vi "niFpgaMemoryEmulationDramWriteAndRequestData.vi"(0 "address":u32, 1 "name":string, 2 "number of elements":u32, 3 "fifo size":u32, 5 "data":i32, 7 "write":bool, 9 "input valid":bool, 11 "error in (no error)":errorcluster, 12 "byte enables":i64, 13 "ref in wired":bool) -> (10 "ready for input":bool, 15 "error out":errorcluster)   [LabVIEW 2017]
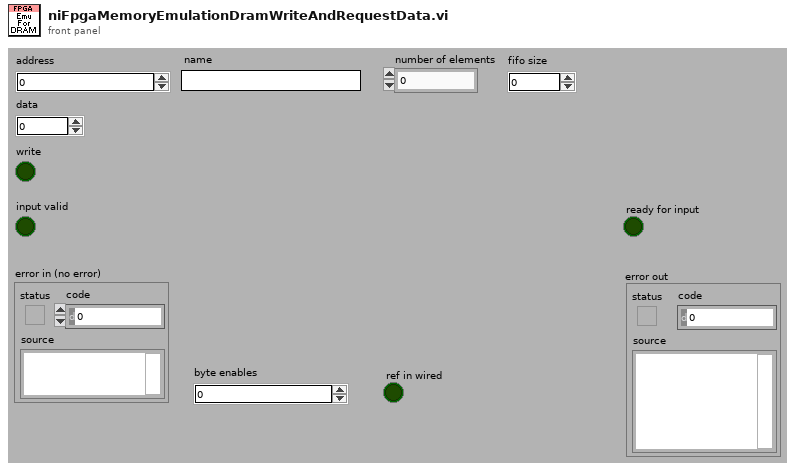
[diagram p1: front panel]
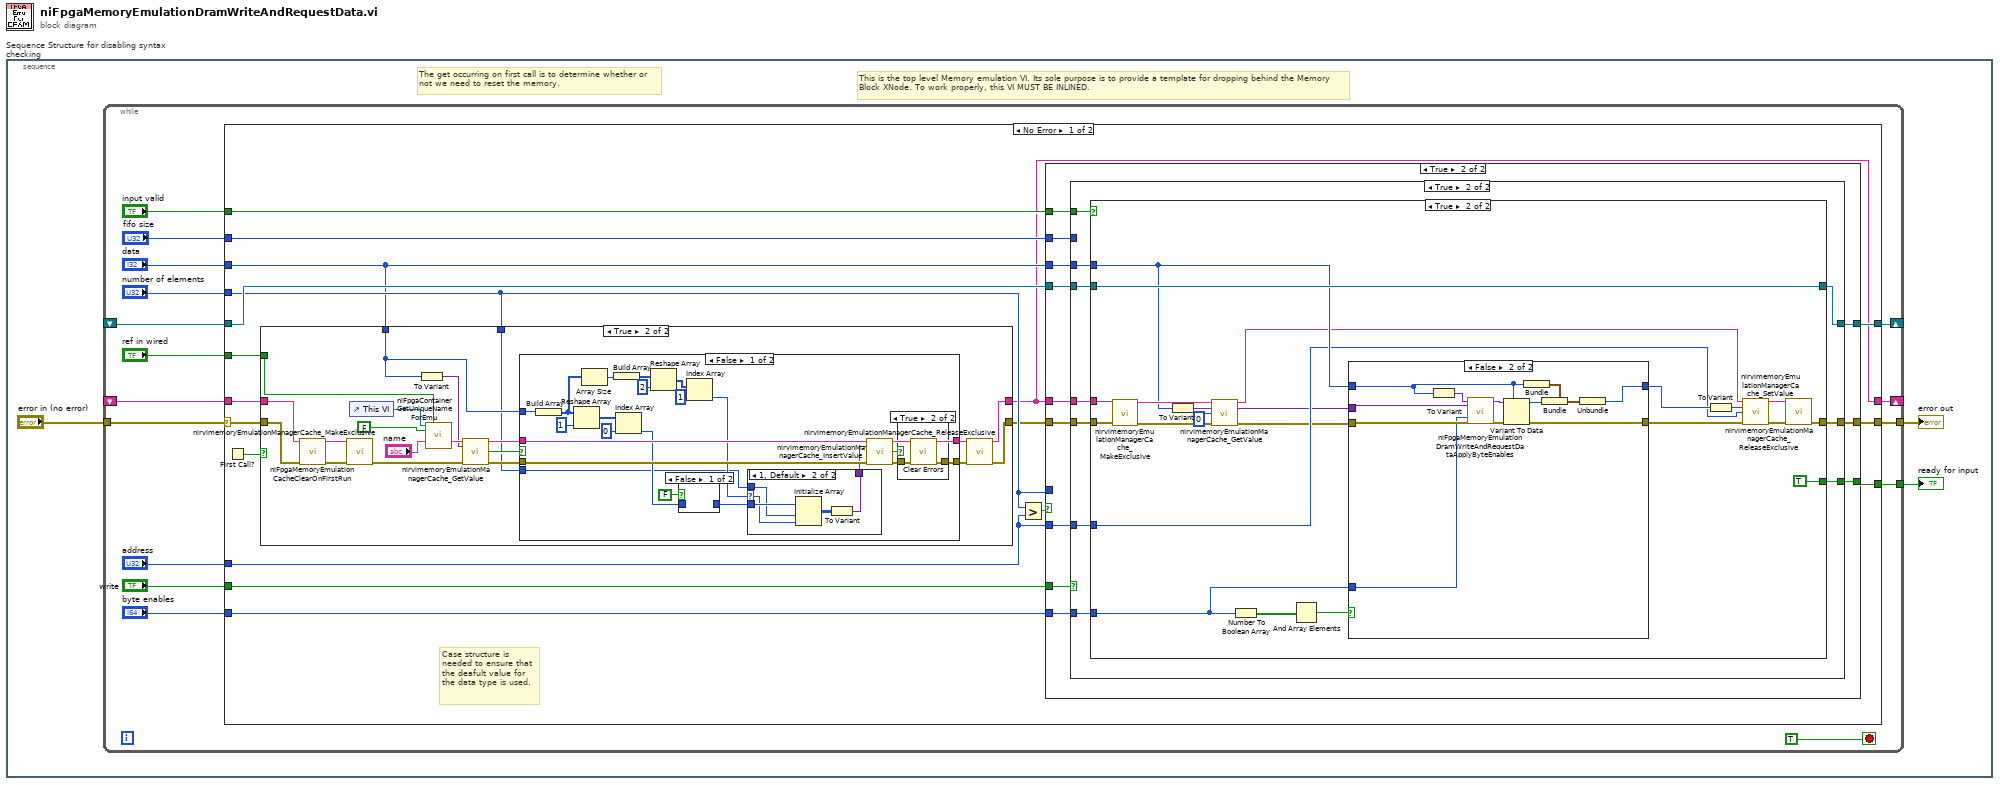
[diagram p0: block diagram]
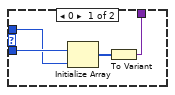
[diagram p3: hidden frame]
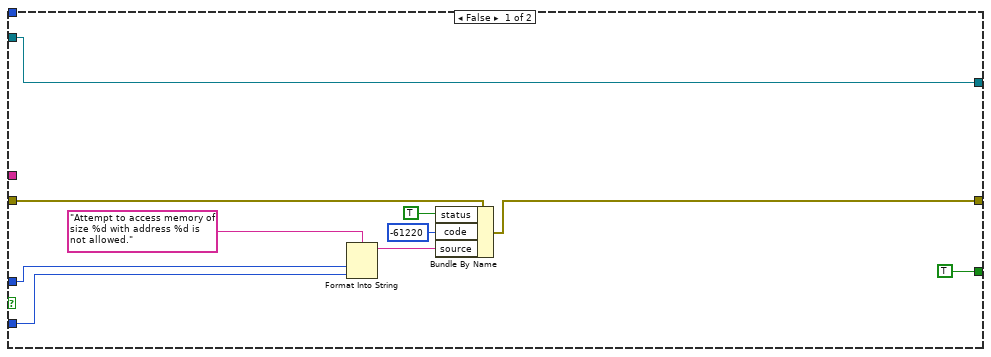
[diagram p7: hidden frame]
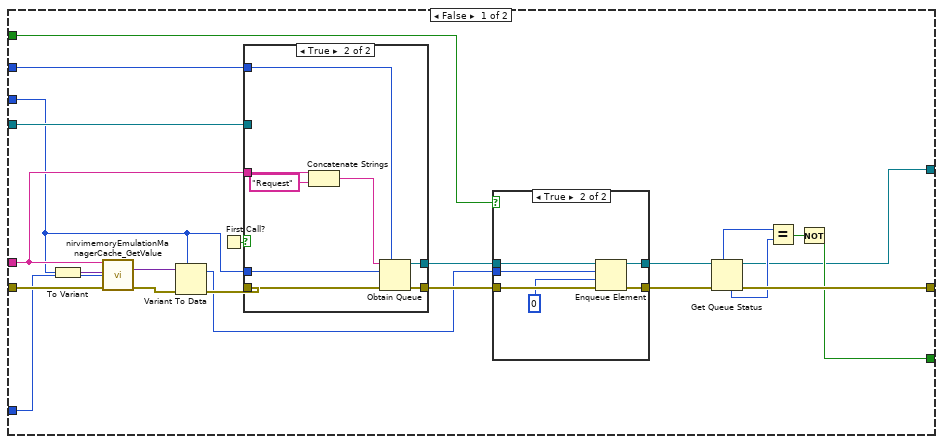
[diagram p8: hidden frame]
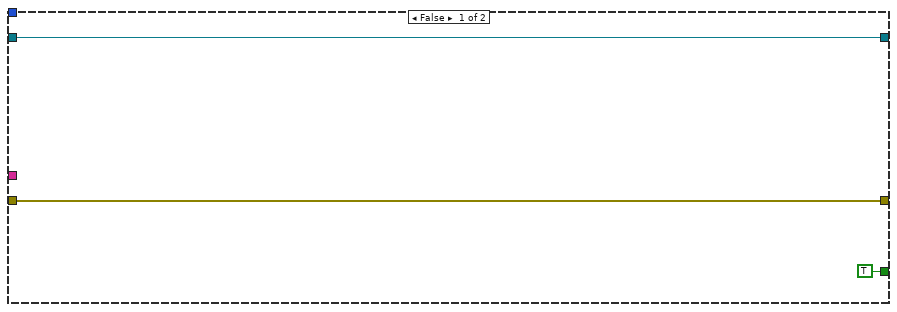
[diagram p11: hidden frame]
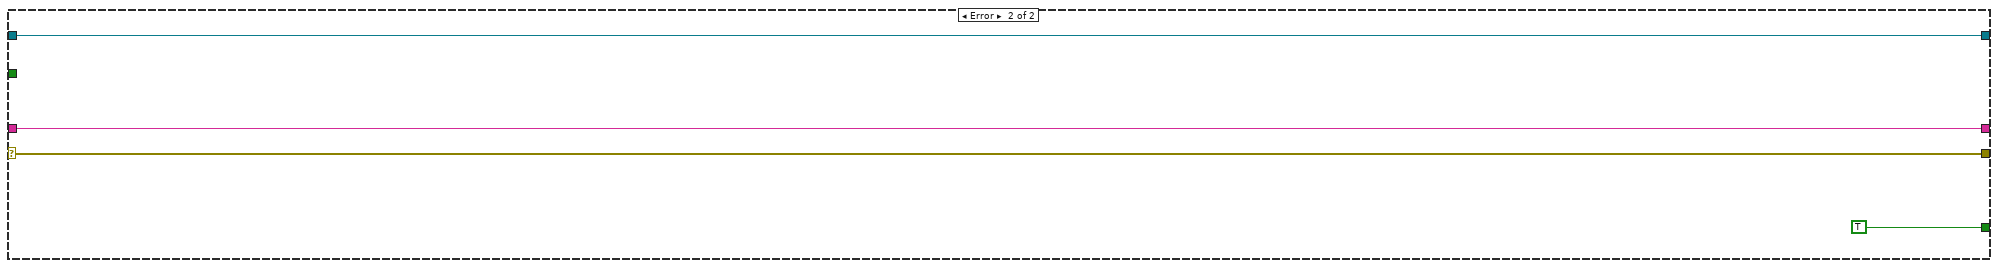
[diagram p13: hidden frame]
diagram:
  n1 = stacked-sequence "Sequence Structure for disabling syntax checking" {
    frame #0 {
      # "The get occurring on first call is to determine whether or not we need to reset the memory."
      # "This is the top level Memory emulation VI. Its sole purpose is to provide a template for dropping behind the Memory Block XNode. To work properly, this VI MUST BE INLINED."
      n2 = while {
        shift-right: [w17] -> _
        shift-left: _ -> [w19]
        tunnel: [w16] -> w1
        tunnel: "error in (no error)" -> [w11]
        tunnel: [w7] -> w3
        shift-right: [w5] -> _
        shift-left: _ -> [w4]
        stop <- TRUE stop-if-true
        n3 = case shown="No Error" w11 {
          selector: w11 -> [w20 w212]
          tunnel: "number of elements" -> [w25 _]
          tunnel: w19 -> [w21 w211]
          tunnel: [w23 w211] -> w17
          tunnel: "write" -> [w36 _]
          tunnel: [w35 w212] -> w16
          tunnel: "address" -> [w37 _]
          tunnel: "data" -> [w24 _]
          tunnel: "ref in wired" -> [w27 _]
          tunnel: "input valid" -> [w31 _]
          tunnel: "byte enables" -> [w34 _]
          tunnel: [w30 TRUE ("ready for input")] -> w7
          tunnel: "fifo size" -> [w33 _]
          tunnel: [w29 w210] -> w5
          tunnel: w4 -> [w28 w210]
          frame No Error {
            # "Case structure is needed to ensure that the deafult value for the data type is used."
            n4 = First Call?() -> (First Call?: T/F=w26:bool)
            n5 = case shown="True" w26 {
              tunnel: w21 -> [w38 w44]
              tunnel: w20 -> [w39 w45]
              tunnel: [w39 w53] -> w22
              tunnel: [w38 w51] -> w23
              tunnel: w27 -> [_ w57]
              tunnel: w25 -> [_ w40]
              tunnel: w24 -> [_ w42]
              frame False {
              }
              frame True {
                n6 = call <vilib>:"niFpgaMemoryEmulationCacheClearOnFirstRun.vi"("Key"=w44, "error in"=w45) -> ("Key (dup)"=w43:string, "error out"=w46:errorcluster)  [unwired: 12 in]
                n7 = call <vilib>:"nirvimemoryEmulationManagerCache_MakeExclusive.vi"("Key"=w43, "error in"=w46) -> ("error out"=w55:errorcluster)  [unwired: 12 in, 1 out]
                n8 = control-ref of="This VI"() -> (w58:refnum<vi>)
                n9 = To Variant(anything=w42) -> (Variant=w41:variant)
                n10 = call <vilib>:"niFpgaContainerGetUniqueNameForEmu.vi"("parent VI"=w58, "ref in wired"=w57, "local"=FALSE, "name in"="name") -> ("name out"=w54:string)  [unwired: 11 in]
                n11 = call <vilib>:"nirvimemoryEmulationManagerCache_GetValue.vi"("Key"=w54, "Value"=w41, "error in (no error)"=w55) -> ("Key"=w48:string, "Found"=w47:bool, "error out"=w49:errorcluster)  [unwired: 9 in, 1 out]
                n12 = case shown="False" w47 {
                  tunnel: w49 -> [w79 w96]
                  tunnel: w48 -> [w78 w95]
                  tunnel: [w77 w96] -> w52
                  tunnel: w42 -> [w72 _]
                  tunnel: [w76 w95] -> w50
                  tunnel: w40 -> [w61 _]
                  frame False {
                    n13 = Build Array(w72) -> (w64:i32[])
                    n14 = Reshape Array(w64, 1 ("dimension size")) -> (w75:i32[])
                    n15 = Array Size(array=w64) -> (size(s)=w65:i32)
                    n16 = Build Array(w65) -> (w67:i32[])
                    n17 = Index Array(array=w75, index=0) -> (element=w70:i32)
                    n18 = Reshape Array(w67, 2 ("dimension size")) -> (w69:i32[])
                    n19 = case shown="False" FALSE {
                      tunnel: w70 -> [_ w91]
                      tunnel: [_ w91] -> w62
                      frame False {
                      }
                      frame True {
                      }
                    }
                    n20 = Index Array(array=w69, index=1) -> (element=w63:i32)
                    n21 = case shown="1, Default" w63 {
                      selector: w63 -> [_ w86]
                      tunnel: w62 -> [w85 w89]
                      tunnel: w61 -> [w84 w87]
                      tunnel: [w82 w90] -> w60
                      frame 0 {
                        n22 = Initialize Array(w85, w84) -> (w83:i32[])
                        n23 = To Variant(anything=w83) -> (Variant=w82:variant)
                      }
                      frame 1, Default {
                        n24 = Initialize Array(w89, w87, w86) -> (w88:i32[][])
                        n25 = To Variant(anything=w88) -> (Variant=w90:variant)
                      }
                    }
                    n26 = call <vilib>:"nirvimemoryEmulationManagerCache_InsertValue.vi"("Key"=w78, "Value"=w60, "error in (no error)"=w79) -> ("Key"=w76:string, "Found"=w81:bool, "error out"=w80:errorcluster)  [unwired: 1 in, 9 out]
                    n27 = case shown="True" w81 {
                      tunnel: w80 -> [w92 w94]
                      tunnel: [w92 w93] -> w77
                      frame False {
                      }
                      frame True {
                        n28 = call <vilib>:"Clear Errors.vi"("error in (no error)"=w94) -> ("error out"=w93:errorcluster)  [unwired: 1 in, 5 out]
                      }
                    }
                  }
                  frame True {
                  }
                }
                n29 = call <vilib>:"nirvimemoryEmulationManagerCache_ReleaseExclusive.vi"("Key"=w50, "error in"=w52) -> ("Key (dup)"=w51:string, "error out"=w53:errorcluster)  [unwired: 12 in]
              }
            }
            n30 = Greater?(x=w25, y=w37) -> (0:w32:bool)
            n31 = case shown="True" w32 {
              tunnel: w24 -> [_ w107]
              tunnel: w37 -> [w104 w108]
              tunnel: w22 -> [w103 w109]
              tunnel: w36 -> [_ w117]
              tunnel: [w102 w118] -> w35
              tunnel: w25 -> [w105 _]
              tunnel: w23 -> [_ w110]
              tunnel: w34 -> [_ w116]
              tunnel: w33 -> [_ w115]
              tunnel: w31 -> [_ w114]
              tunnel: [TRUE ("ready for input") w113] -> w30
              tunnel: [w97 w112] -> w29
              tunnel: w28 -> [w97 w111]
              frame False {
                n32 = Format Into String(format string="Attempt to access memory of size %d with address %d is not allowed." ("error message (\"\")"), w105, w104) -> (resulting string=w99:string)  [unwired: 2 in, 1 out]
                n33 = Bundle By Name(cluster=w103, "status"=TRUE, "code"=-61220, "source"=w99) -> (w102:errorcluster)
              }
              frame True {
                n34 = case shown="True" w117 {
                  tunnel: w108 -> [w121 w164]
                  tunnel: [w135 w160] -> w118
                  tunnel: w109 -> [w124 w161]
                  tunnel: w116 -> [_ w169]
                  tunnel: w110 -> [w127 w162]
                  tunnel: w115 -> [w122 _]
                  tunnel: w114 -> [w138 w168]
                  tunnel: [w131 w167] -> w113
                  tunnel: [w130 w165] -> w112
                  tunnel: w111 -> [w126 w166]
                  tunnel: w107 -> [w119 w163]
                  frame False {
                    n35 = To Variant(anything=w119) -> (Variant=w123:variant)
                    n36 = call <vilib>:"nirvimemoryEmulationManagerCache_GetValue.vi"("Key"=w127, "Value"=w123, "Address"=w121, "error in (no error)"=w124) -> ("Value"=w128:variant, "error out"=w129:errorcluster)  [unwired: 10 out]
                    n37 = Variant To Data(error in=w129, type=w119, Variant=w128) -> (data=w120:i32, error out=w125:errorcluster)
                    n38 = First Call?() -> (First Call?: T/F=w141:bool)
                    n39 = case shown="True" w141 {
                      tunnel: w125 -> [w150 w159]
                      tunnel: w127 -> [_ w154]
                      tunnel: w122 -> [_ w158]
                      tunnel: [w150 w157] -> w140
                      tunnel: [w151 w156] -> w139
                      tunnel: w126 -> [w151 _]
                      tunnel: w119 -> [_ w155]
                      frame False {
                      }
                      frame True {
                        n40 = Concatenate Strings(w154, "Request" ("string")) -> (w152:string)
                        n41 = Obtain Queue(max queue size (-1, unlimited)=w158, name (unnamed)=w152, element data type=w155, error in (no error)=w159) -> (queue out=w156:refnum<queue>, error out=w157:errorcluster)  [unwired: 1 in, 1 out]
                      }
                    }
                    n42 = case shown="True" w138 {
                      tunnel: w140 -> [w143 w149]
                      tunnel: w139 -> [w142 w148]
                      tunnel: [w142 w147] -> w136
                      tunnel: [w143 w146] -> w137
                      tunnel: w120 -> [_ w144]
                      frame False {
                      }
                      frame True {
                        n43 = Enqueue Element(queue=w148, element=w144, timeout in ms (-1)=0, error in (no error)=w149) -> (queue out=w147:refnum<queue>, error out=w146:errorcluster)  [unwired: 1 out]
                      }
                    }
                    n44 = Get Queue Status(queue=w136, error in (no error)=w137) -> (queue out=w130:refnum<queue>, max queue size=w134:i32, error out=w135:errorcluster, # elements in queue=w133:i32)  [unwired: 1 in, 4 out]
                    n45 = Equal?(x=w134, y=w133) -> (x = y?=w132:bool)
                    n46 = Not(x=w132) -> (.not. x?=w131:bool)
                  }
                  frame True {
                    n47 = case shown="True" w168 {
                      tunnel: w164 -> [_ w179]
                      tunnel: [w171 w185] -> w160
                      tunnel: w169 -> [_ w173]
                      tunnel: w161 -> [w171 w187]
                      tunnel: w162 -> [_ w188]
                      tunnel: [TRUE ("ready for input") TRUE ("ready for input")] -> w167
                      tunnel: w166 -> [w170 w192]
                      tunnel: [w170 w192] -> w165
                      tunnel: w163 -> [_ w182]
                      frame False {
                      }
                      frame True {
                        n48 = call <vilib>:"nirvimemoryEmulationManagerCache_MakeExclusive.vi"("Key"=w188, "error in"=w187) -> ("Key (dup)"=w189:string, "error out"=w190:errorcluster)  [unwired: 12 in]
                        n49 = To Variant(anything=w182) -> (Variant=w183:variant)
                        n50 = call <vilib>:"nirvimemoryEmulationManagerCache_GetValue.vi"("Key"=w189, "Value"=w183, "Address"=0, "error in (no error)"=w190) -> ("Key"=w178:string, "Value"=w177:variant, "error out"=w176:errorcluster)  [unwired: 9 out]
                        n51 = Number To Boolean Array(number=w173) -> (Boolean array=w175:bool[])
                        n52 = And Array Elements(Boolean array=w175) -> (logical AND=w174:bool)
                        n53 = case shown="False" w174 {
                          tunnel: [w195 w208] -> w191
                          tunnel: [w196 w197] -> w180
                          tunnel: w182 -> [w196 w199]
                          tunnel: w177 -> [_ w204]
                          tunnel: w176 -> [w195 w203]
                          tunnel: w173 -> [_ w202]
                          frame True {
                            # "111111111111111...1"
                            # "Every byte is enabled so we can bypass the logic required to emulate byte enable functionality."
                          }
                          frame False {
                            n54 = To Variant(anything=w199) -> (Variant=w207:variant)
                            n55 = call <vilib>:"niFpgaMemoryEmulationDramWriteAndRequestDataApplyByteEnables.vi"("New Value"=w207, "Current Value"=w204, "Byte Enables"=w202, "error in (no error)"=w203) -> ("Byte Enabled Value"=w205:variant, "error out"=w206:errorcluster)  [unwired: 14 in]
                            n56 = Variant To Data(error in=w206, type=w199, Variant=w205) -> (data=w200:i32, error out=w208:errorcluster)
                            n57 = Bundle("data"=w199) -> (w198:cluster{"data":i32})  [unwired: 1 in]
                            n58 = Bundle(cluster=w198, "data"=w200) -> (w201:cluster{"data":i32})
                            n59 = Unbundle(w201) -> ("data"=w197:i32)
                          }
                        }
                        n60 = To Variant(anything=w180) -> (Variant=w194:variant)
                        n61 = call <vilib>:"nirvimemoryEmulationManagerCache_SetValue.vi"("Key"=w178, "Value"=w194, "Address"=w179, "error in (no error)"=w191) -> ("Key"=w184:string, "error out"=w186:errorcluster)  [unwired: 10 out]
                        n62 = call <vilib>:"nirvimemoryEmulationManagerCache_ReleaseExclusive.vi"("Key"=w184, "error in"=w186) -> ("error out"=w185:errorcluster)  [unwired: 12 in, 1 out]
                      }
                    }
                  }
                }
              }
            }
          }
          frame Error {
          }
        }
      }
      "error out" <- w1
      "ready for input" <- w3
    }
  }
